vi "Get Metrics.vi"(8 "error in (no error)":errorcluster, 9 "Coerce (T)":bool=TRUE, 10 "Finger Positions":T2={"Thumb"=[0.0, 0.0, 0.0], "Middle"=[0.0, 0.0, 0.0], "Index"=[0.0, 0.0, 0.0]}, 11 "MF3 in":refnum<class "MF3.lvclass">) -> (0 "error out":errorcluster, 2 "metrics":T1, 3 "MF3 out":refnum<class "MF3.lvclass">)   [LabVIEW 2011, in "MF3.lvclass"]
uses:
  MF3.lvclass
  controls/Vector3D Fingers.ctl
  MF3.lvclass/MF3.ctl
  <vilib>/Analysis/_algsub.llb/Real Vector Norm.vi
  <vilib>/Analysis/NI_AALPro.lvlib
  <vilib>/ptbypt/NI_PtbyPt.lvlib
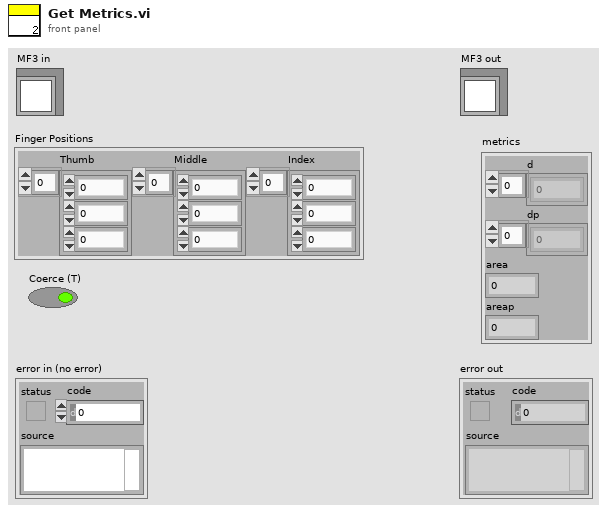
[diagram p1: front panel]
types:
  T1 = cluster{"d":dbl[], "dp":dbl[], "area":dbl, "areap":dbl}
  T2 = typedef "Vector3D Fingers.ctl" = cluster{"Thumb":dbl[], "Middle":dbl[], "Index":dbl[]}
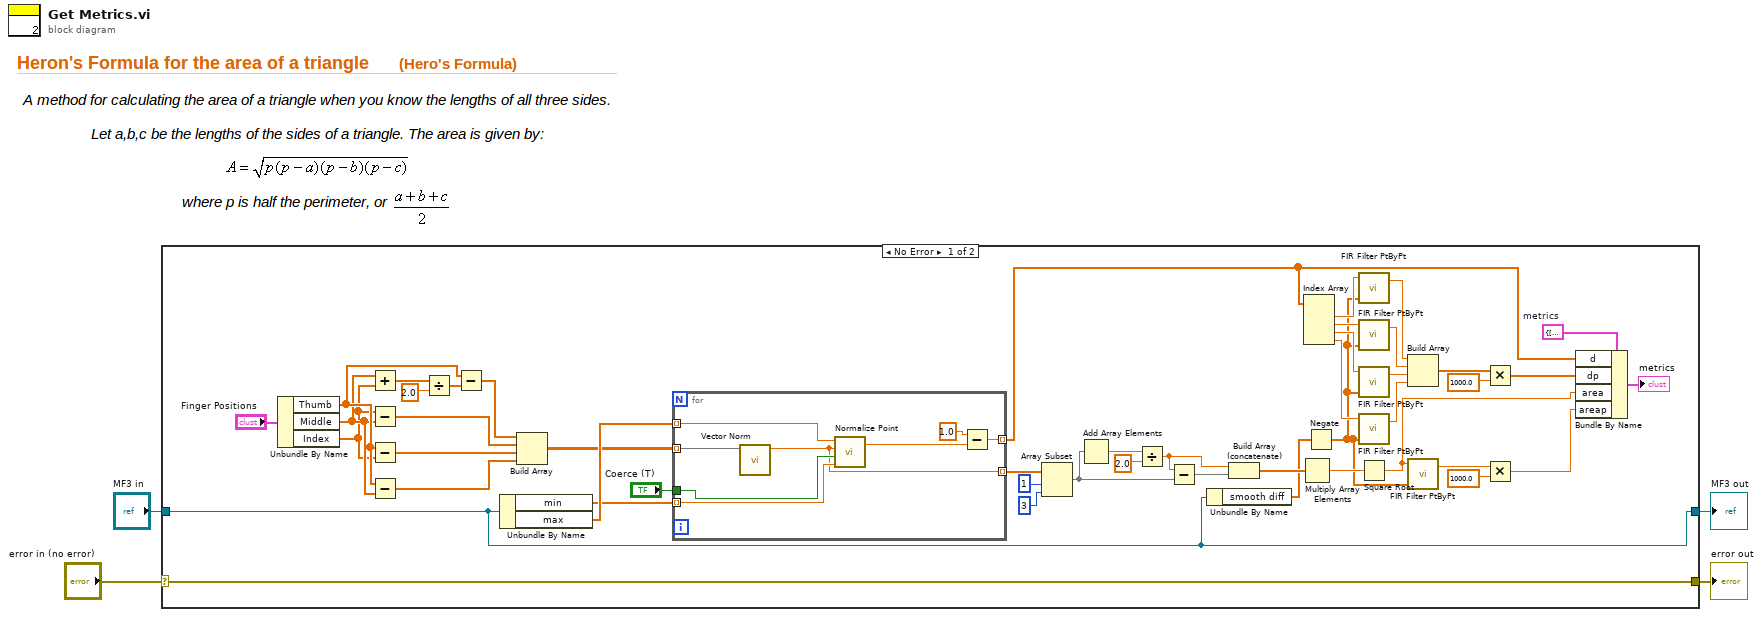
[diagram p0: block diagram]
diagram:
  n1 = case shown="No Error" "error in (no error)" {
    selector: "error in (no error)" -> [w51 w61]
    tunnel: [w51 w61] -> w3
    tunnel: [w23 w60] -> w1
    tunnel: "MF3 in" -> [w23 w60]
    frame No Error {
      w26 = T1 {"d"=[], "dp"=[], "area"=0.0, "areap"=0.0}  # metrics
      n2 = Unbundle By Name("Finger Positions") -> ("Thumb"=w38:dbl[], "Middle"=w37:dbl[], "Index"=w36:dbl[])
      n3 = Add(x=w37, y=w36) -> (x+y=w50:dbl[])
      n4 = Subtract(x=w36, y=w37) -> (x-y=w42:dbl[])
      n5 = Subtract(x=w38, y=w36) -> (x-y=w40:dbl[])
      n6 = Subtract(x=w38, y=w37) -> (x-y=w39:dbl[])
      n7 = Divide(x=w50, y=2.0) -> (x/y=w48:dbl[])
      n8 = Subtract(x=w38, y=w48) -> (x-y=w43:dbl[])
      n9 = Unbundle By Name(w23) -> ("min"=w44:dbl[], "max"=w45:dbl[])
      n10 = Build Array(w43, w42, w40, w39) -> (w41:dbl[][])
      n11 = for {
        tunnel: "Coerce (T)" -> [w59]
        tunnel: [w53] -> w5 mode=indexing
        tunnel: w45 -> [w58] mode=indexing
        tunnel: w44 -> [w57] mode=indexing
        tunnel: w41 -> [w56] mode=indexing
        tunnel: [w52] -> w18 mode=indexing
        n12 = call-poly <vilib>:"Vector Norm.vi"("Input Vector"=w56) -> ("norm"=w52:dbl)  [unwired: 9 in, 1 out]
        n13 = call "Normalize Point.vi"("xmax"=w58, "x"=w52, "Coerce (T)"=w59, "xmin"=w57) -> ("y"=w54:dbl)  [unwired: 2 in]
        n14 = Subtract(x=1.0, y=w54) -> (x-y=w53:dbl)
      }
      n15 = Array Subset(array=w18, index=1, length=3) -> (w31:dbl[])
      n16 = Add Array Elements(numeric array=w31) -> (sum=w33:dbl)
      n17 = Divide(x=w33, y=2.0) -> (x/y=w29:dbl)
      n18 = Subtract(x=w29, y=w31) -> (x-y=w28:dbl[])
      n19 = Unbundle By Name(w23) -> ("smooth diff"=w22:dbl[])
      n20 = Build Array (concatenate)(w29, w28) -> (w27:dbl[])
      n21 = Multiply Array Elements(1:w27) -> (0:w30:dbl)
      n22 = Index Array(array=w5) -> (element #1=w17:dbl, element #2=w14:dbl, element #3=w13:dbl, element #4=w12:dbl)  [unwired: 4 in]
      n23 = Negate(x=w22) -> (-x=w6:dbl[])
      n24 = call <vilib>:"FIR Filter PtByPt.vi"("Forward Coefficients"=w6, "x"=w17) -> ("Filtered x"=w15:dbl)  [unwired: 2 in, 1 out]
      n25 = call <vilib>:"FIR Filter PtByPt.vi"("Forward Coefficients"=w6, "x"=w14) -> ("Filtered x"=w9:dbl)  [unwired: 2 in, 1 out]
      n26 = call <vilib>:"FIR Filter PtByPt.vi"("Forward Coefficients"=w6, "x"=w13) -> ("Filtered x"=w8:dbl)  [unwired: 2 in, 1 out]
      n27 = call <vilib>:"FIR Filter PtByPt.vi"("Forward Coefficients"=w6, "x"=w12) -> ("Filtered x"=w7:dbl)  [unwired: 2 in, 1 out]
      n28 = Square Root(x=w30) -> (sqrt(x)=w24:dbl)
      n29 = Build Array(w15, w9, w8, w7) -> (w11:dbl[])
      n30 = call <vilib>:"FIR Filter PtByPt.vi"("Forward Coefficients"=w6, "x"=w24) -> ("Filtered x"=w21:dbl)  [unwired: 2 in, 1 out]
      n31 = Multiply(x=w11, y=1000.0) -> (x*y=w10:dbl[])
      n32 = Multiply(x=w21, y=1000.0) -> (x*y=w20:dbl)
      n33 = Bundle By Name(cluster=w26, "d"=w5, "dp"=w10, "area"=w24, "areap"=w20) -> (→"metrics":T1)
    }
    frame Error {
    }
  }
  "error out" <- w3
  "MF3 out" <- w1
